vi "GetImpairReports.vi"(8 "error in (no error)":errorcluster, 11 "C37PmuImpairPlugin":refnum<class "C37PMUImpairPlugin.lvclass">) -> (0 "error out":errorcluster, 3 "C37PmuImpairPlugin":refnum<class "C37PMUImpairPlugin.lvclass">)   [LabVIEW 2014, in "PmuImpairPlugins.lvlib" / "C37PMUImpairPlugin.lvclass"]
uses:
  C37PMUImpairPlugin.lvclass
  PmuImpairPluginBase_class/PmuImpairPluginBase.lvclass/PmuImpairPluginBase.ctl
  EventPlugins/EventPluginBaseClass/TypeDefs/clEvtReport.ctl
  PmuImpairPluginBase_class/Accessors/Read dblEventSignalArray.vi
  PmuImpairPluginBase_class/Accessors/Read clEvtConfig.vi
  PmuImpairPluginBase_class/Accessors/Read BusNumber.vi
  PmuImpairPluginBase_class/Accessors/Read clImpairConfig.vi
  PmuImpairPluginBase_class/Accessors/Read dblImpairParams.vi
  EventPlugins/EventPluginBaseClass/EventPluginBaseClass.lvclass
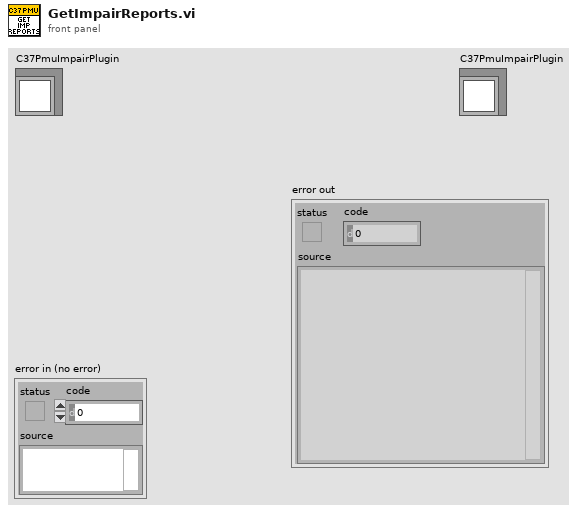
[diagram p1: front panel]
types:
  T1 = typedef "EventPlugins.lvlib/EventPluginBaseClass.lvclass/clEvtReport.ctl" = cluster{"Timestamp":dbl, "Synx":cdb[], "Freq":dbl, "ROCOF":dbl, "ID":i16}
  T2 = typedef "PmuImpairPlugins.lvlib/PmuImpairPluginBase.lvclass/clImpairConfig.ctl" = cluster{"FilterType":string, "bPosSeq":bool}
  T3 = typedef "EventPlugins.lvlib/EventPluginBaseClass.lvclass/dblEvtSignalArray.ctl" = dbl[][]
  T4 = typedef "EventPlugins.lvlib/EventPluginBaseClass.lvclass/clEvtReportArray.ctl" = T1[]
  T5 = typedef "EventPlugins.lvlib/EventPluginBaseClass.lvclass/clEvtConfig.ctl" = cluster{"T0(UTC)":dbl, "F0":dbl, "Fs":i32, "FSamp":u32, "bPosSeq":bool}
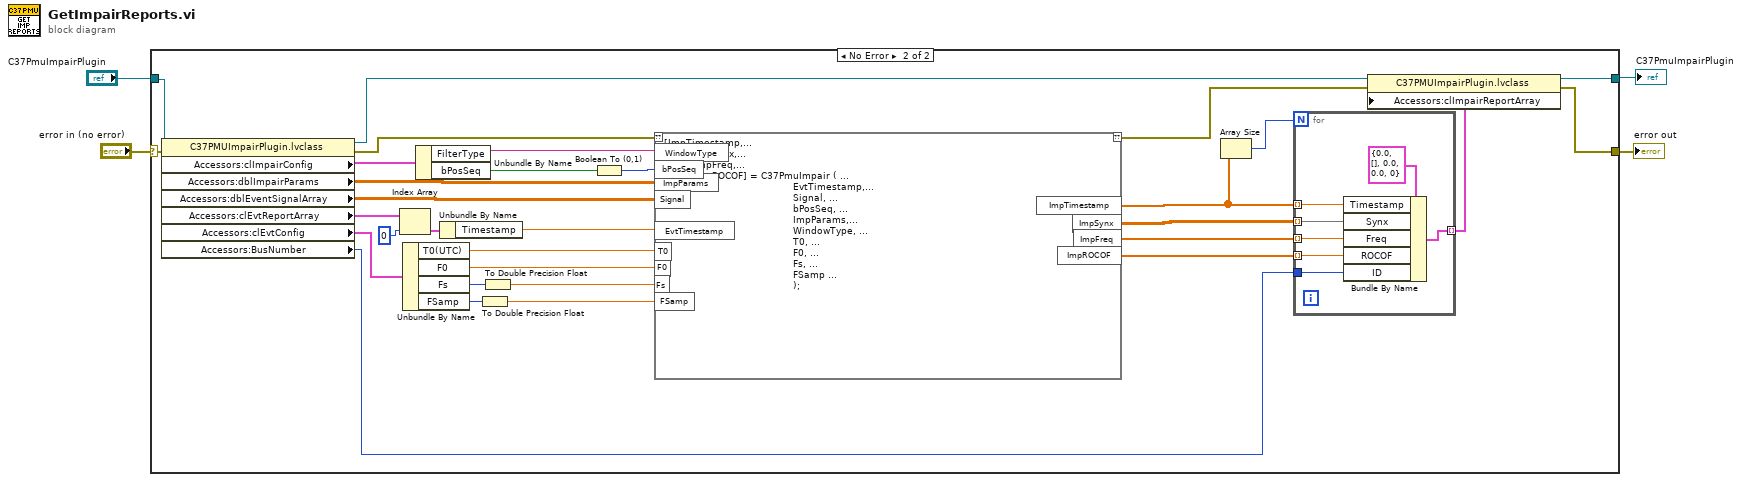
[diagram p0: block diagram]
diagram:
  n1 = case shown="No Error" "error in (no error)" {
    selector: "error in (no error)" -> [w6 w32]
    tunnel: [w5 w35] -> w1
    tunnel: "C37PmuImpairPlugin" -> [w5 w33]
    tunnel: [w6 w34] -> w2
    frame Error {
    }
    frame No Error {
      n2 = property class="C37PMUImpairPlugin.lvclass"(reference=w33, error in=w32) -> (reference out=w31:refnum<class "C37PMUImpairPlugin.lvclass">, error out=w23:errorcluster, "Accessors:clImpairConfig"=w25:T2, "Accessors:dblImpairParams"=w26:dbl[][], "Accessors:dblEventSignalArray"=w22:T3, "Accessors:clEvtReportArray"=w21:T4, "Accessors:clEvtConfig"=w17:T5, "Accessors:BusNumber"=w8:u8)
      n3 = Index Array(array=w21, index=0) -> (element=w19:T1)
      n4 = Unbundle By Name(w17) -> ("T0(UTC)"=w16:dbl, "F0"=w15:dbl, "Fs"=w14:i32, "FSamp"=w13:u32)
      n5 = Unbundle By Name(w25) -> ("FilterType"=w10:string, "bPosSeq"=w9:bool)
      n6 = Unbundle By Name(w19) -> ("Timestamp"=w18:dbl)
      n7 = To Double Precision Float(number=w13) -> (double precision float=w11:dbl)
      n8 = To Double Precision Float(number=w14) -> (double precision float=w12:dbl)
      n9 = Boolean To (0,1)(Boolean=w9) -> (0, 1=w7:i16)
      n10 = script code="[ImpTimestamp,...\n          ImpSynx,...\n          ImpFreq,...\n          ImpROCOF] = C37PmuImpair ( ...\n                                           EvtTimestamp,...\n                                           Signal, ... \n                                           bPosSeq, ...    \n                                           ImpParams,...\n                                           WindowType, ...\n                                           T0, ...\n                                           F0, ...\n                                           Fs, ...\n                                           FSamp ...\n                                           );"("??"=w23, "ImpParams"=w26, "WindowType"=w10, "bPosSeq"=w7, "F0"=w15, "Fs"=w12, "FSamp"=w11, "EvtTimestamp"=w18, "Signal"=w22, "T0"=w16) -> ("??"=w28:errorcluster, "ImpTimestamp"=w30:dbl[], "ImpSynx"=w27:cdb[][], "ImpFreq"=w37:dbl[], "ImpROCOF"=w36:dbl[])
      n11 = Array Size(array=w30) -> (size(s)=w29:i32)
      n12 = for {
        N: w29 -> [_]
        tunnel: w30 -> [w44] mode=indexing
        tunnel: w37 -> [w43] mode=indexing
        tunnel: w36 -> [w42] mode=indexing
        tunnel: w27 -> [w41] mode=indexing
        tunnel: [w39] -> w24 mode=indexing
        tunnel: w8 -> [w38]
        n13 = Bundle By Name(cluster=T1 {"Timestamp"=0.0, "Synx"=[], "Freq"=0.0, "ROCOF"=0.0, "ID"=0} ("clEvtReport"), "Timestamp"=w44, "Synx"=w41, "Freq"=w43, "ROCOF"=w42, "ID"=w38) -> (w39:T1)
      }
      n14 = property class="C37PMUImpairPlugin.lvclass"(reference=w31, error in=w28, "Accessors:clImpairReportArray"=w24) -> (reference out=w35:refnum<class "C37PMUImpairPlugin.lvclass">, error out=w34:errorcluster)
    }
  }
  "error out" <- w2
  "C37PmuImpairPlugin" <- w1
